vi "cblas idamax.vi"(5 "n":i32=-1, 7 "incx":i32=1, 11 "x":dbl[](array[numeric])) -> (0 "error":i32, 3 "idamax":i32)   [LabVIEW 2017, in "NI_AALBLAS.lvlib"]
doc: "Decimates input sequence <B>X</B> by <B>incX</B> and returns the index of the element in the decimated sequence with the greatest absolute value. The data type you wire to the <B>X</B> input determines the polymorphic instance to use."
uses:
  NI_AALBLAS.lvlib
  <resource>/lvblas.dll
panel:
  # "long cblas_idamax(n, *x, incx)"
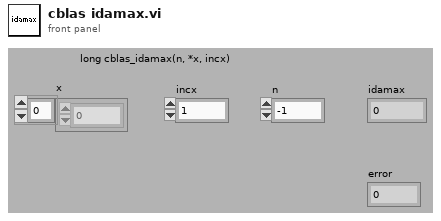
[diagram p1: front panel]
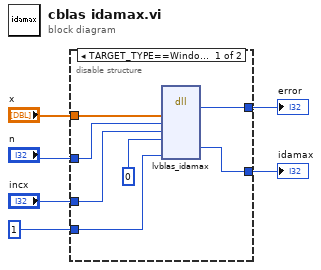
[diagram p0: block diagram]
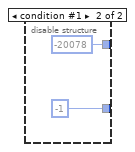
[diagram p2: hidden frame]
diagram:
  n1 = disable-structure shown="TARGET_TYPE==Windows||TARGET_TYPE==Unix||TARGET_TYPE==Mac||TARGET_TYPE==RT" {
    disable-tunnel: "x" -> [w12 _]
    disable-tunnel: "n" -> [w11 _]
    disable-tunnel: "incx" -> [w10 _]
    disable-tunnel: [w8 -1] -> w3
    disable-tunnel: [w13 -20078] -> w2
    disable-tunnel: 1 -> [w7 _]
    frame condition #0 (active) {
      n2 = dll-call lib="C:/Program Files (x86)/National Instruments/LabVIEW 2017/resource/lvblas.*" fn="lvblas_idamax" ("LVBLAS.dll:BLASVectorMaxH")("X"=w12, "N"=w11, "IncX"=w10, "startX"=0, "check"=w7) -> ("error"=w13:i32, "maxindex"=w8:i32)  [unwired: 8 in, 3 out]
    }
    frame condition #1 {
    }
  }
  "idamax" <- w3
  "error" <- w2
